vi "FPGA_TypeConversionTest.vi"() -> ()   [LabVIEW 2014]
uses:
  <vilib>/rvi/Emulation/niFpgaGetClockAttributes.vi
  <vilib>/rvi/Emulation/niFpgaSctlEmulationGetInTimedLoop.vi
  <vilib>/rvi/Emulation/niFpgaEmulationReportErrorSimple.vi
  <vilib>/rvi/Emulation/niFpgaCriticalErrorInLSC.vi
panel:
  in  "stop":bool
  out "s? t:f":i16
  out "Waveform Chart":i16(graph)
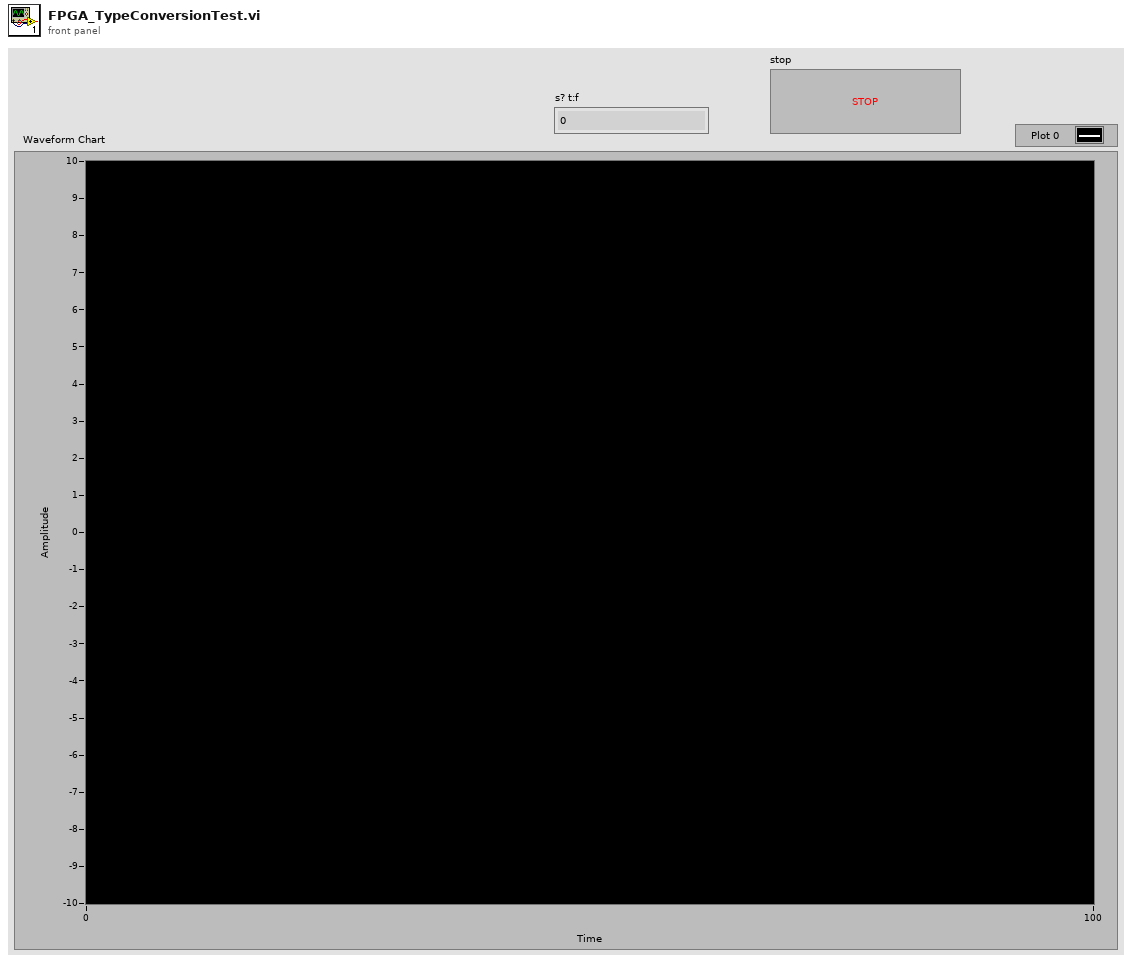
[diagram p1: front panel]
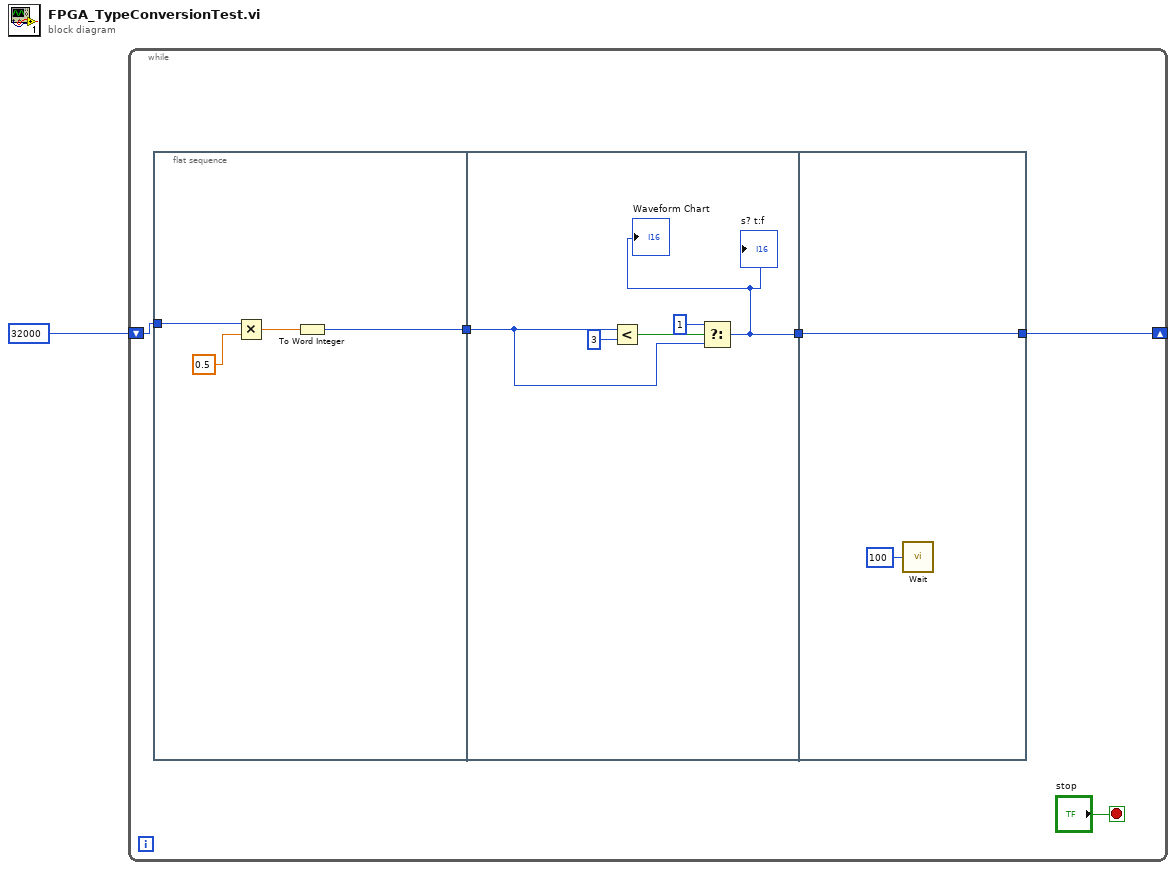
[diagram p0: block diagram]
diagram:
  n1 = while {
    shift-right: [w4] -> _
    shift-left: i16 32000 -> [w6]
    stop <- "stop" stop-if-true
    n2 = flat-sequence {
      tunnel: w6 -> [w10]
      tunnel: [w7] -> w5
      tunnel: w5 -> [w13]
      tunnel: [w11] -> w3
      tunnel: [w17] -> w4
      tunnel: w3 -> [w17]
      frame #0 {
        n3 = Multiply(x=w10, y=sgl 0.5) -> (x*y=w8:sgl)
        n4 = To Word Integer(number=w8) -> (16bit integer=w7:i16)
      }
      frame #1 {
        n5 = Less?(x=w13, y=i16 3) -> (x < y?=w14:bool)
        n6 = Select(t=i16 1, s=w14, f=w13) -> (s? t:f=w11:i16)
        "Waveform Chart" <- w11
        "s? t:f" <- w11
      }
      frame #2 {
        n7 = call "Wait"("Count(mSec)"=u32 100) -> ()  [unwired: 1 out]
      }
    }
  }
